vi "renezvous example 1.vi"() -> ()   [LabVIEW 2020]
panel:
  in  "Boolean":bool
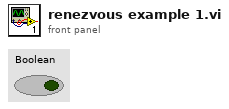
[diagram p1: front panel]
types:
  T1 = typedef "Rendezvous RefNum" = refnum<k1>
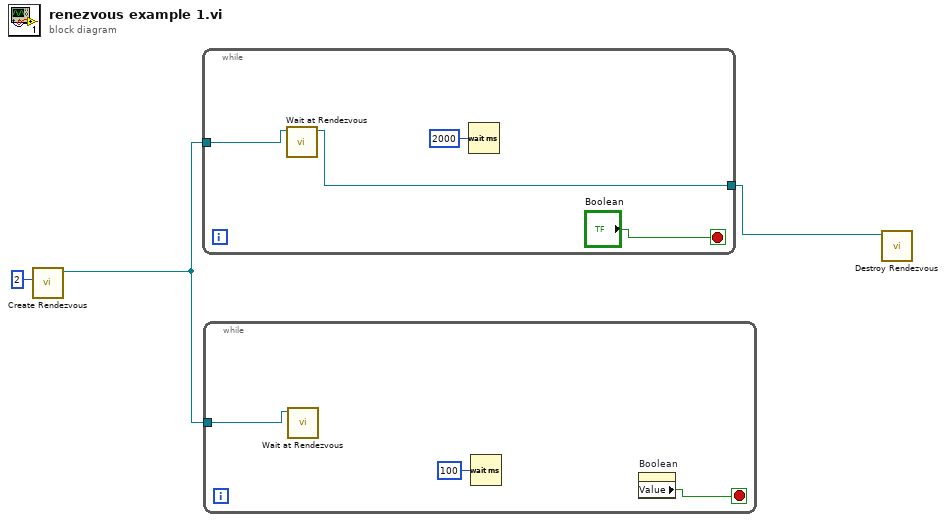
[diagram p0: block diagram]
diagram:
  n1 = call <vilib>:"Create Rendezvous.vi"("size (2)"=2) -> ("rendezvous"=w2:T1)  [unwired: 4 in, 2 out]
  n2 = while {
    tunnel: w2 -> [w7]
    tunnel: [w5] -> w1
    stop <- "Boolean" stop-if-true
    n3 = call <vilib>:"Wait at Rendezvous.vi"("rendezvous"=w7) -> ("rendezvous out"=w5:T1)  [unwired: 4 in, 2 out]
    n4 = Wait (ms)(milliseconds to wait=u32 2000) -> ()  [unwired: 1 out]
  }
  n5 = while {
    tunnel: w2 -> [w10]
    stop <- w8 stop-if-true
    n6 = call <vilib>:"Wait at Rendezvous.vi"("rendezvous"=w10) -> ()  [unwired: 4 in, 3 out]
    n7 = Wait (ms)(milliseconds to wait=u32 100) -> ()  [unwired: 1 out]
    n8 = property on="Boolean" class="Bool (strict)"() -> ("Value"=w8:bool)  [unwired: 2 in, 2 out]
  }
  n9 = call <vilib>:"Destroy Rendezvous.vi"("rendezvous"=w1) -> ()  [unwired: 5 in, 2 out]
